vi "Resources.vi"() -> (3 "Resources":refnum<class "VisaResource.lvclass">[](array[class]))   [LabVIEW 2020, in "RP2040.lvlib" / "RP2040Platform.lvclass"]
uses:
  RP2040Platform.lvclass
  Builds/picoG/ppl/PicoG-Core.lvlibp/PicoG-Processor/PicoG-Core/VisaResource/VisaResource.lvclass
  <vilib>/Instr/_visa.llb/VISA Find Search Mode.ctl
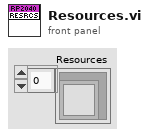
[diagram p1: front panel]
types:
  T1 = typedef "VISA Find Search Mode.ctl" = u32
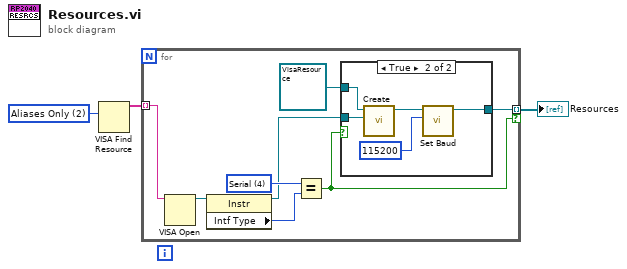
[diagram p0: block diagram]
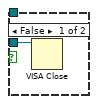
[diagram p2: hidden frame]
diagram:
  w3 = T1 2 items=["Canonical Names Only"=0, "Aliases Only"=2, "Include Matching Aliases"=3, "Include All Aliases"=4] ("Search Mode")
  n1 = VISA Find Resource(10:w3) -> (3:w2:string[])  [unwired: 2 in, 2 out]
  n2 = for {
    tunnel: w2 -> [w11] mode=indexing
    tunnel: [w5] -> w1 mode=indexing if=w7
    w9 = u16 4 items=["GPIB"=1, "VXI"=2, "GPIB-VXI"=3, "Serial"=4, "PXI"=5, "TCPIP"=6, "USB"=7, "FireWire"=9] ("Interface Information:Interface Type")
    n3 = VISA Open(VISA resource name=w11) -> (VISA resource name=w10:refnum<visa-resource-name>)  [unwired: 4 in, 1 out]
    n4 = property class="Instr"(reference=w10) -> (reference out=w6:refnum<visa-resource-name>, "Intf Type"=w8:u16)  [unwired: 1 in, 1 out]
    n5 = Equal?(x=w9, y=w8) -> (x = y?=w7:bool)
    n6 = case shown="True" w7 {
      tunnel: w6 -> [w12 w17]
      tunnel: [_ w14] -> w5
      tunnel: refnum<class "VisaResource.lvclass"> refnum ("PicoG-Core:VisaResource.lvclass") -> [_ w16]
      frame False {
        n7 = VISA Close(VISA resource name=w12) -> ()  [unwired: 1 in, 1 out]
      }
      frame True {
        n8 = call-dynamic "Create.vi"("Resource"=w17, "VisaResource in"=w16) -> ("VisaResource out"=w15:refnum<class "VisaResource.lvclass">)  [unwired: 8 in, 1 out]
        n9 = call "Set Baud.vi"("Baud (115200)"=u32 115200, "VisaResource in"=w15) -> ("VisaResource out"=w14:refnum<class "VisaResource.lvclass">)  [unwired: 8 in, 1 out]
      }
    }
  }
  "Resources" <- w1
